vi "Controller Board Temp.vi"(8 "Error In":errorcluster, 9 "Line In Voltage":dbl=10.0, 10 "Power Supply In":string="PowerSupply", 11 "DMM In":string="DMM") -> (0 "Error Out":errorcluster, 3 "Temperature":dbl)   [LabVIEW 2015]
doc: "After applying maximum voltage and maximum ambient temperature, measure the temperature of the controller board."
uses:
  <instrlib>/Driver Simulation/Fixture/EnvironmentSettings.ctl
  <instrlib>/Driver Simulation/DMM/TemperatureSensorTypes.ctl
  <instrlib>/Driver Simulation/Fixture.lvlib
  <instrlib>/Driver Simulation/Power Supply.lvlib
  <instrlib>/Driver Simulation/DMM.lvlib
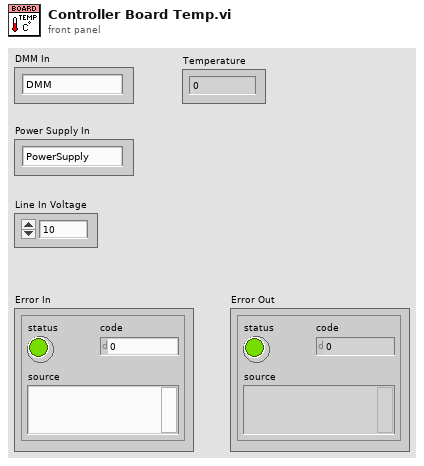
[diagram p1: front panel]
types:
  T1 = typedef "Driver Simulation.lvlib/DMM.lvlib/TemperatureSensorTypes.ctl" = i32
  T2 = typedef "Driver Simulation.lvlib/Fixture.lvlib/EnvironmentSettings.ctl" = enum16{"Temperature", "Light Intensity"}
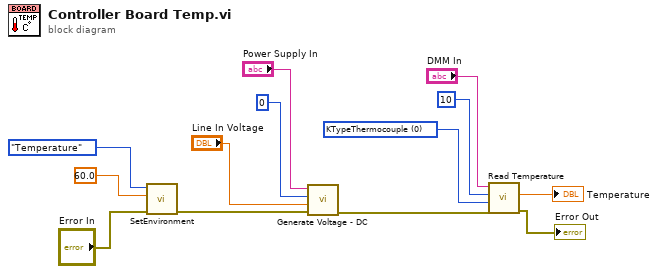
[diagram p0: block diagram]
diagram:
  w4 = T1 0 items=["KTypeThermocouple", "JTypeThermocouple"] ("Sensor Type")
  n1 = call <instrlib>:"SetEnvironment.vi"("error in (no error)"="Error In", "Value"=60.0, "Setting"=EnvironmentSettings."Temperature") -> ("error out"=w13:errorcluster)  [unwired: 8 in]
  n2 = call <instrlib>:"Generate Voltage - DC.vi"("error in (no error)"=w13, "Output Voltage"="Line In Voltage", "Channel"=0, "Power Supply in"="Power Supply In") -> ("error out"=w12:errorcluster)  [unwired: 6 in, 1 out]
  n3 = call <instrlib>:"Read Temperature.vi"("error in (no error)"=w12, "Sensor Type"=w4, "Channel"=10, "DMM in"="DMM In") -> ("error out"=→"Error Out":errorcluster, "Temperature (C)"=→"Temperature":dbl)  [unwired: 5 in, 1 out]
